vi "EI-1050 Example.vi"() -> (0 "error out":errorcluster)   [LabVIEW 2020]
panel:
  in  "Read Names":string[](array[string])=["SBUS0_TEMP", "SBUS0_RH"]
  out "Read Values":dbl[](array[numeric]) format="%.2f"
  out "ErrorAddress (Reads)":i32
  in  "Update Interval (ms)":u32=1000
  in  "stop":bool
  in  "Config Values":dbl[](array[numeric])=[0.0, 1.0, 2.0] format="%.2f"
  in  "Config Names":string[](array[string])=["SBUS_ALL_POWER_DIONUM", "SBUS0_DATA_DIONUM", "SBUS0_CLOCK_DIONUM"]
  out "Error String":string
  out "ConnectionType Out":i32=3
  out "DeviceType Out":i32=7
  in  "Identifier":string="LJM_idANY"
  in  "ConnectionType":string="LJM_ctANY"
  in  "DeviceType":string="LJM_dtANY"
  out "ErrorAddress":i32
  # "By default this example configures one sensor as SBUS0\nDefault Wiring Configs:\n    Power(Red): DIO0\n    Ground(Black): GND\n    Data(Green): DIO1\n    Clock(White): DIO2\n    Enable(Brown): not connected"
  # "Note: the SBUS temp registers return temperature in Kelvin"
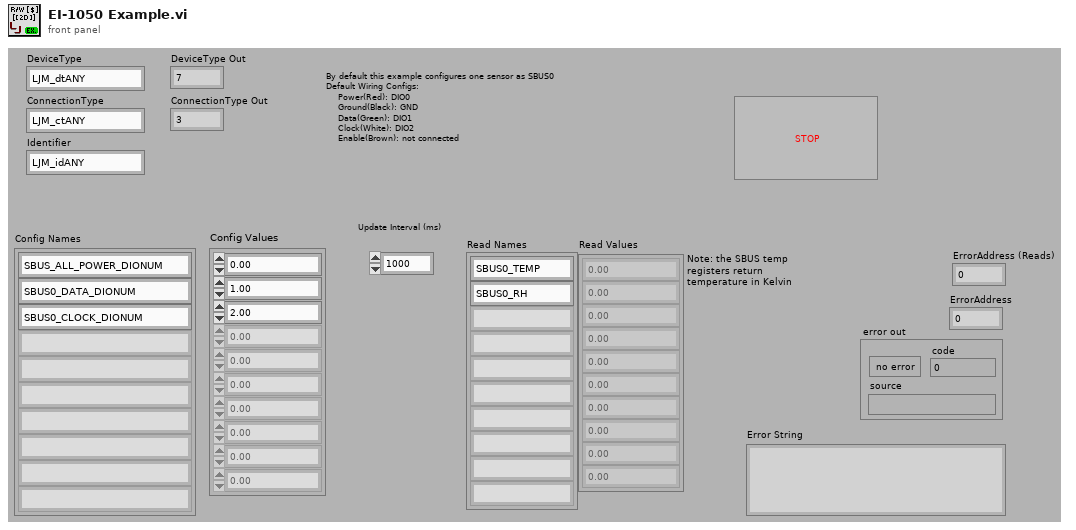
[diagram p1: front panel]
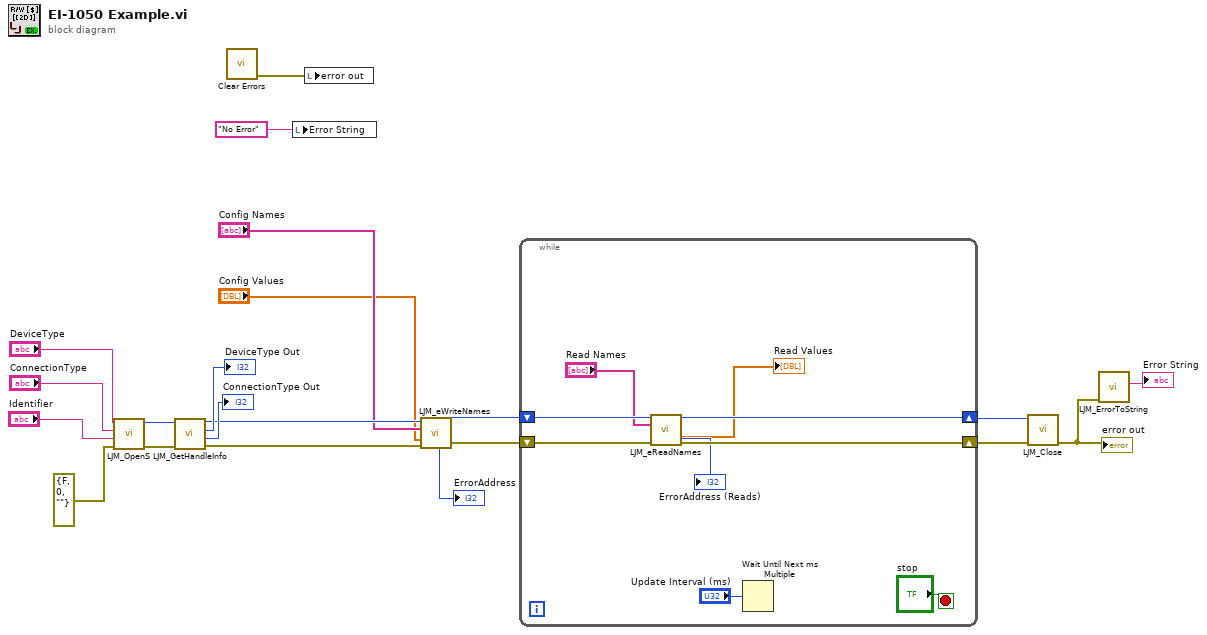
[diagram p0: block diagram]
diagram:
  n1 = call "LJM_OpenS.vi"("error in"=errorcluster {"status"=FALSE, "code"=0, "source"=""} ("error in (no error)"), "Identifier"="Identifier", "ConnectionType"="ConnectionType", "DeviceType"="DeviceType") -> ("error out"=w20:errorcluster, "Handle"=w19:i32)  [unwired: 6 in]
  n2 = call "LJM_GetHandleInfo.vi"("error in"=w20, "Handle In"=w19) -> ("error out"=w8:errorcluster, "ConnectionType"=→"ConnectionType Out":i32, "DeviceType"=→"DeviceType Out":i32, "Handle Out"=w11:i32)  [unwired: 2 in, 4 out]
  n3 = call <vilib>:"Clear Errors.vi"() -> ("error out"=w1:errorcluster)  [unwired: 6 in, 1 out]
  n4 = local write "Error String"("No Error" ("Error String")) -> ()
  n5 = local write "error out"(w1) -> ()
  n6 = call "LJM_eWriteNames.vi"("Handle In"=w11, "aNames"="Config Names", "aValuesIn"="Config Values", "error in"=w8) -> ("Handle Out"=w6:i32, "ErrorAddress"=→"ErrorAddress":i32, "error out"=w5:errorcluster)  [unwired: 9 in]
  n7 = while {
    shift-right: [w26] -> w4
    shift-left: w6 -> [w28]
    shift-right: [w25] -> w3
    shift-left: w5 -> [w27]
    stop <- "stop" stop-if-true
    n8 = call "LJM_eReadNames.vi"("Handle In"=w28, "aNames"="Read Names", "error in"=w27) -> ("Handle Out"=w26:i32, "aValuesOut"=→"Read Values":dbl[], "ErrorAddress"=→"ErrorAddress (Reads)":i32, "error out"=w25:errorcluster)  [unwired: 9 in]
    n9 = Wait Until Next ms Multiple(millisecond multiple="Update Interval (ms)") -> ()  [unwired: 1 out]
  }
  n10 = call "LJM_Close.vi"("error in"=w3, "Handle"=w4) -> ("error out"=w13:errorcluster)  [unwired: 9 in]
  "error out" <- w13
  n11 = call "LJM_ErrorToString.vi"("error in"=w13) -> ("String"=→"Error String":string)  [unwired: 10 in]
